vi "Deadband.vi"(9 "Deadband":dbl, 10 "Value 2":dbl, 11 "Value":dbl) -> (2 "Within Deadband?":bool)   [LabVIEW 2019]
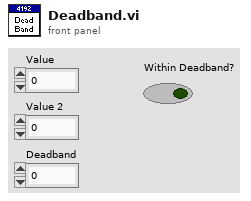
[diagram p1: front panel]
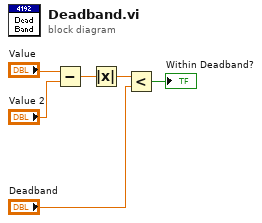
[diagram p0: block diagram]
diagram:
  n1 = Subtract(x="Value", y="Value 2") -> (x-y=w4:dbl)
  n2 = Absolute Value(x=w4) -> (abs(x)=w3:dbl)
  n3 = Less?(x=w3, y="Deadband") -> (x < y?=→"Within Deadband?":bool)
